vi "FMDLCloseKeithley2450-old.vi"(1 "error in (no error)":errorcluster, 2 "VISA resource name":refnum<visa-resource-name>) -> (0 "error out":errorcluster)   [LabVIEW 2018]
uses:
  <instrlib>/Keithley 2450/Keithley 2450.lvlib
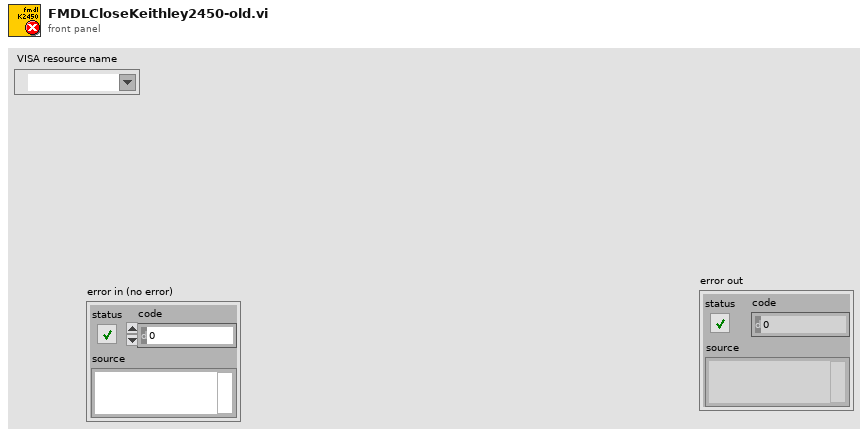
[diagram p1: front panel]
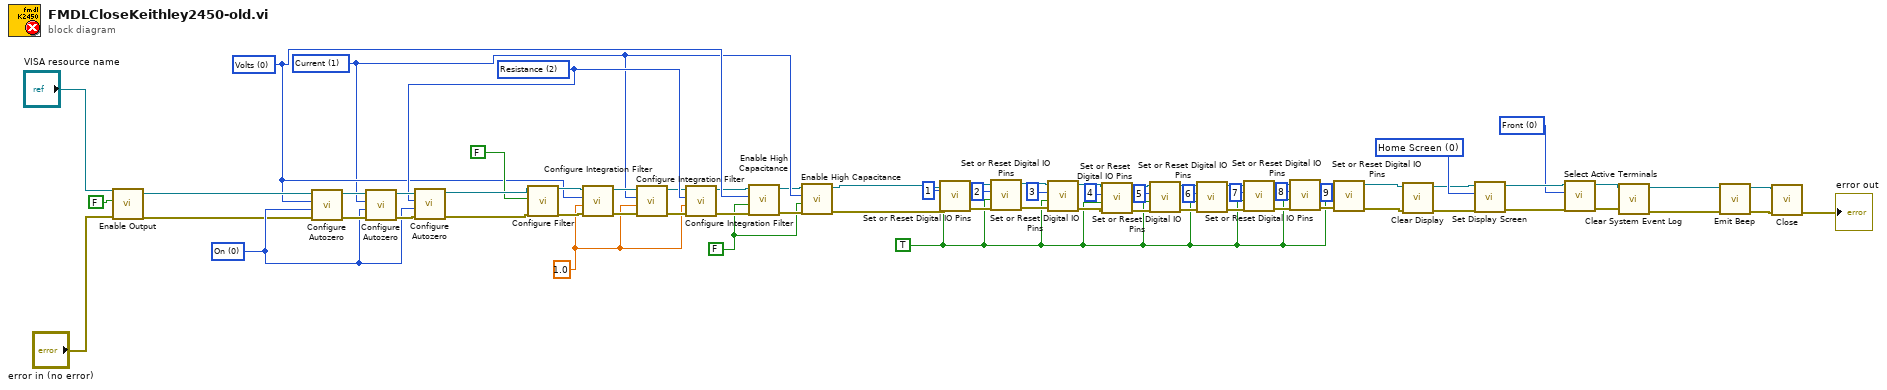
[diagram p0: block diagram]
diagram:
  w5 = u16 0 items=["Front", "Rear"] ("Active Terminals (0: Front)")
  w14 = u16 0 items=["Home Screen", "Source Screen", "Plot Screen", "User-defined Screen", "Statistics Screen", "Settings Screen", "Graph Screen", "Data sheet Screen"] ("Screen Home")
  w21 = TRUE ("Digital IO Line (T: Bit High)")
  w43 = FALSE ("Enable High Capacitance (T:Enable)")
  w50 = 1.0 ("Measurement Speed (1 PLC)")
  w53 = u16 2 items=["Volts", "Current", "Resistance"] ("Function (0: Volts)")
  w48 = u16 1 items=["Volts", "Current", "Resistance"] ("Function (0: Volts)")
  w67 = u16 0 items=["On", "Off"] ("Autozero  (0: On)")
  w49 = u16 0 items=["Volts", "Current", "Resistance"] ("Function (0: Volts)")
  n1 = call <instrlib>:"Enable Output.vi"("error in (no error)"="error in (no error)", "Enable Output (T: Enable)"=FALSE, "VISA resource name"="VISA resource name") -> ("error out"=w61:errorcluster, "VISA resource name out"=w63:refnum<visa-resource-name>)  [unwired: 7 in]
  n2 = call <instrlib>:"Configure Autozero.vi"("error in (no error)"=w61, "Autozero  (0: On)"=w67, "Function (0: Volts)"=w49, "VISA resource name"=w63) -> ("error out"=w70:errorcluster, "VISA resource name out"=w71:refnum<visa-resource-name>)  [unwired: 6 in]
  n3 = call <instrlib>:"Configure Autozero.vi"("error in (no error)"=w70, "Autozero  (0: On)"=w67, "Function (0: Volts)"=w48, "VISA resource name"=w71) -> ("error out"=w68:errorcluster, "VISA resource name out"=w69:refnum<visa-resource-name>)  [unwired: 6 in]
  n4 = call <instrlib>:"Configure Autozero.vi"("error in (no error)"=w68, "Autozero  (0: On)"=w67, "Function (0: Volts)"=w53, "VISA resource name"=w69) -> ("error out"=w59:errorcluster, "VISA resource name out"=w60:refnum<visa-resource-name>)  [unwired: 6 in]
  n5 = call <instrlib>:"Configure Filter.vi"("VISA resource name"=w60, "Enable Filter  (T: Enable)"=FALSE, "error in (no error)"=w59) -> ("VISA resource name out"=w57:refnum<visa-resource-name>, "error out"=w56:errorcluster)  [unwired: 15 in]
  n6 = call <instrlib>:"Configure Integration Filter.vi"("error in (no error)"=w56, "Measurement Speed (1 PLC)"=w50, "Function (0: Volts)"=w49, "VISA resource name"=w57) -> ("error out"=w54:errorcluster, "VISA resource name out"=w55:refnum<visa-resource-name>)  [unwired: 6 in]
  n7 = call <instrlib>:"Configure Integration Filter.vi"("error in (no error)"=w54, "Measurement Speed (1 PLC)"=w50, "Function (0: Volts)"=w48, "VISA resource name"=w55) -> ("error out"=w51:errorcluster, "VISA resource name out"=w52:refnum<visa-resource-name>)  [unwired: 6 in]
  n8 = call <instrlib>:"Configure Integration Filter.vi"("error in (no error)"=w51, "Measurement Speed (1 PLC)"=w50, "Function (0: Volts)"=w53, "VISA resource name"=w52) -> ("error out"=w46:errorcluster, "VISA resource name out"=w47:refnum<visa-resource-name>)  [unwired: 6 in]
  n9 = call <instrlib>:"Enable High Capacitance.vi"("error in (no error)"=w46, "Enable High Capacitance (T:Enable)"=w43, "Function (0: Volts)"=w49, "VISA resource name"=w47) -> ("error out"=w44:errorcluster, "VISA resource name out"=w45:refnum<visa-resource-name>)  [unwired: 6 in]
  n10 = call <instrlib>:"Enable High Capacitance.vi"("error in (no error)"=w44, "Enable High Capacitance (T:Enable)"=w43, "Function (0: Volts)"=w48, "VISA resource name"=w45) -> ("error out"=w41:errorcluster, "VISA resource name out"=w42:refnum<visa-resource-name>)  [unwired: 6 in]
  n11 = call <instrlib>:"Set or Reset Digital IO Pins.vi"("error in (no error)"=w41, "Digital IO Line (T: Bit High)"=w21, "Digital IO Line (1)"=u32 1, "VISA resource name"=w42) -> ("error out"=w38:errorcluster, "VISA resource name out"=w39:refnum<visa-resource-name>)  [unwired: 6 in]
  n12 = call <instrlib>:"Set or Reset Digital IO Pins.vi"("error in (no error)"=w38, "Digital IO Line (T: Bit High)"=w21, "Digital IO Line (1)"=u32 2, "VISA resource name"=w39) -> ("error out"=w35:errorcluster, "VISA resource name out"=w36:refnum<visa-resource-name>)  [unwired: 6 in]
  n13 = call <instrlib>:"Set or Reset Digital IO Pins.vi"("error in (no error)"=w35, "Digital IO Line (T: Bit High)"=w21, "Digital IO Line (1)"=u32 3, "VISA resource name"=w36) -> ("error out"=w32:errorcluster, "VISA resource name out"=w33:refnum<visa-resource-name>)  [unwired: 6 in]
  n14 = call <instrlib>:"Set or Reset Digital IO Pins.vi"("error in (no error)"=w32, "Digital IO Line (T: Bit High)"=w21, "Digital IO Line (1)"=u32 4, "VISA resource name"=w33) -> ("error out"=w30:errorcluster, "VISA resource name out"=w31:refnum<visa-resource-name>)  [unwired: 6 in]
  n15 = call <instrlib>:"Set or Reset Digital IO Pins.vi"("error in (no error)"=w30, "Digital IO Line (T: Bit High)"=w21, "Digital IO Line (1)"=u32 5, "VISA resource name"=w31) -> ("error out"=w28:errorcluster, "VISA resource name out"=w29:refnum<visa-resource-name>)  [unwired: 6 in]
  n16 = call <instrlib>:"Set or Reset Digital IO Pins.vi"("error in (no error)"=w28, "Digital IO Line (T: Bit High)"=w21, "Digital IO Line (1)"=u32 6, "VISA resource name"=w29) -> ("error out"=w26:errorcluster, "VISA resource name out"=w27:refnum<visa-resource-name>)  [unwired: 6 in]
  n17 = call <instrlib>:"Set or Reset Digital IO Pins.vi"("error in (no error)"=w26, "Digital IO Line (T: Bit High)"=w21, "Digital IO Line (1)"=u32 7, "VISA resource name"=w27) -> ("error out"=w24:errorcluster, "VISA resource name out"=w25:refnum<visa-resource-name>)  [unwired: 6 in]
  n18 = call <instrlib>:"Set or Reset Digital IO Pins.vi"("error in (no error)"=w24, "Digital IO Line (T: Bit High)"=w21, "Digital IO Line (1)"=u32 8, "VISA resource name"=w25) -> ("error out"=w22:errorcluster, "VISA resource name out"=w23:refnum<visa-resource-name>)  [unwired: 6 in]
  n19 = call <instrlib>:"Set or Reset Digital IO Pins.vi"("error in (no error)"=w22, "Digital IO Line (T: Bit High)"=w21, "Digital IO Line (1)"=u32 9, "VISA resource name"=w23) -> ("error out"=w1:errorcluster, "VISA resource name out"=w2:refnum<visa-resource-name>)  [unwired: 6 in]
  n20 = call <instrlib>:"Clear Display.vi"("error in (no error)"=w1, "VISA resource name"=w2) -> ("error out"=w3:errorcluster, "VISA resource name out"=w4:refnum<visa-resource-name>)  [unwired: 8 in]
  n21 = call <instrlib>:"Set Display Screen.vi"("error in (no error)"=w3, "Screen Home"=w14, "VISA resource name"=w4) -> ("error out"=w6:errorcluster, "VISA resource name out"=w7:refnum<visa-resource-name>)  [unwired: 7 in]
  n22 = call <instrlib>:"Select Active Terminals.vi"("error in (no error)"=w6, "Active Terminals (0: Front)"=w5, "VISA resource name"=w7) -> ("error out"=w8:errorcluster, "VISA resource name out"=w9:refnum<visa-resource-name>)  [unwired: 7 in]
  n23 = call <instrlib>:"Clear System Event Log.vi"("error in (no error)"=w8, "VISA resource name"=w9) -> ("error out"=w10:errorcluster, "VISA resource name out"=w11:refnum<visa-resource-name>)  [unwired: 8 in]
  n24 = call <instrlib>:"Emit Beep.vi"("error in (no error)"=w10, "VISA resource name"=w11) -> ("error out"=w13:errorcluster, "VISA resource name out"=w12:refnum<visa-resource-name>)  [unwired: 8 in]
  n25 = call <instrlib>:"Close.vi"("error in (no error)"=w13, "VISA resource name"=w12) -> ("error out"=→"error out":errorcluster)  [unwired: 9 in]
